vi "Iso Measurement Read.vi"(8 "error in":errorcluster, 11 "Iso Measurement in":refnum<class "Iso Measurement.lvclass">) -> (0 "error out":errorcluster, 1 "Changed or First Call?":bool, 2 "Iso Measurement ACT":bool, 3 "Iso Measurement out":refnum<class "Iso Measurement.lvclass">)   [LabVIEW 2023, in "Iso Measurement.lvclass"]
uses:
  Iso Measurement.lvclass
  fe525089-57de-4ef3-b309-4dcf5b94c711.vi
  <vilib>/ADAS Replay HIL/Channels/Tag Wrapper/Tag Wrapper.lvlib
  <vilib>/ADAS Replay HIL/Channels/Tag Wrapper/Polymorphic/Read Channel (Boolean).vi
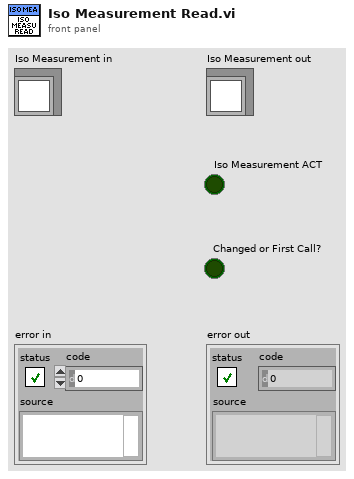
[diagram p1: front panel]
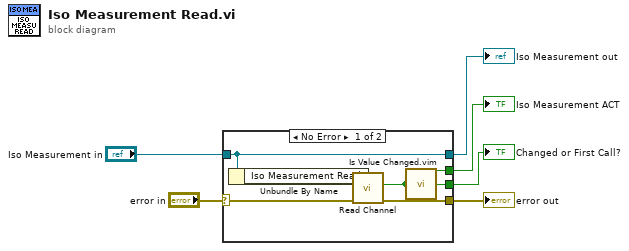
[diagram p0: block diagram]
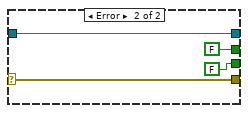
[diagram p2: hidden frame]
diagram:
  n1 = case shown="No Error" "error in" {
    selector: "error in" -> [w11 w16]
    tunnel: [w10 w16] -> w5
    tunnel: [w9 w15] -> w3
    tunnel: "Iso Measurement in" -> [w9 w15]
    tunnel: [w8 FALSE ("changed or first call?")] -> w2
    tunnel: [w7 FALSE ("Value out")] -> w1
    frame No Error {
      n2 = Unbundle By Name(w9) -> ("Iso Measurement Read"=w12:refnum<k21>)
      n3 = call-poly <vilib>:"Read Channel.vi"("error in"=w11, "ADAS HIL Channel in"=w12) -> ("error out"=w10:errorcluster, "Value out"=w7:bool)  [unwired: 6 in, 2 out]
      n4 = call "Is Value Changed.vim"("value"=w7) -> ("changed or first call?"=w8:bool)
    }
    frame Error {
    }
  }
  "error out" <- w5
  "Iso Measurement out" <- w3
  "Iso Measurement ACT" <- w1
  "Changed or First Call?" <- w2
